vi "CreateExperimentRunNode.vi"(8 "Error In":errorcluster, 10 "Experiment Run":T1, 11 "DOM Document In":refnum<k20>) -> (0 "Error out":errorcluster, 2 "Experiment Run Node":refnum<k20>, 3 "DOM Document Out":refnum<k20>)   [LabVIEW 2012]
uses:
  ExperimentRun.ctl
  ExperimentRunTiming.ctl
  ExperimentRunDose.ctl
  ExperimentRunFluence.ctl
  ExperimentRunTotalCharge.ctl
  <resource>/objmgr/DOMUserDefRef.rc
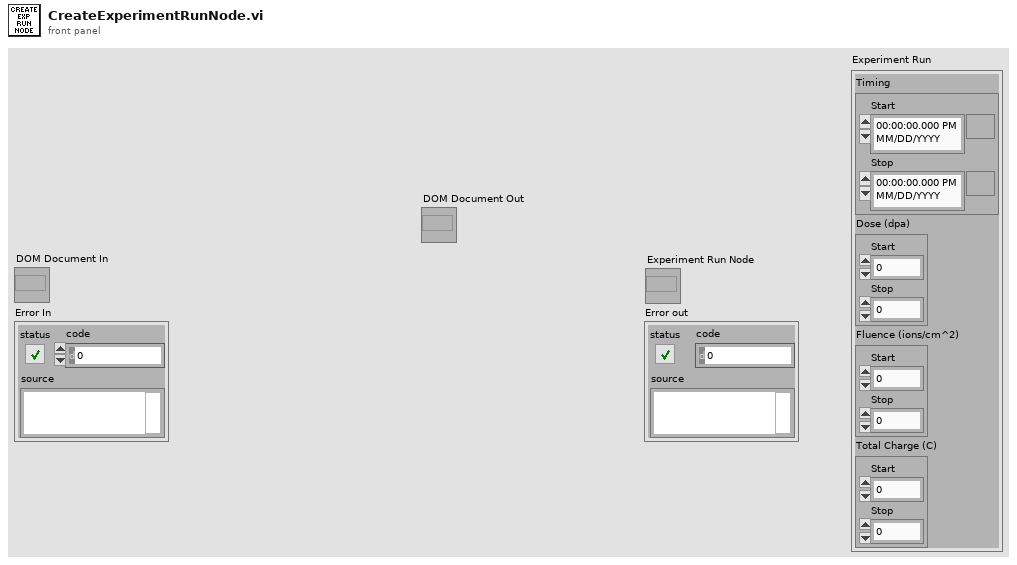
[diagram p1: front panel]
types:
  T1 = typedef "ExperimentRun.ctl" = cluster{"Timing":T2, "Dose (dpa)":T3, "Fluence (ions/cm^2)":T4, "Total Charge (C)":T5}
  T2 = typedef "ExperimentRunTiming.ctl" = cluster{"Start":timestamp, "Stop":timestamp}
  T3 = typedef "ExperimentRunDose.ctl" = cluster{"Start":dbl, "Stop":dbl}
  T4 = typedef "ExperimentRunFluence.ctl" = cluster{"Start":dbl, "Stop":dbl}
  T5 = typedef "ExperimentRunTotalCharge.ctl" = cluster{"Start":dbl, "Stop":dbl}
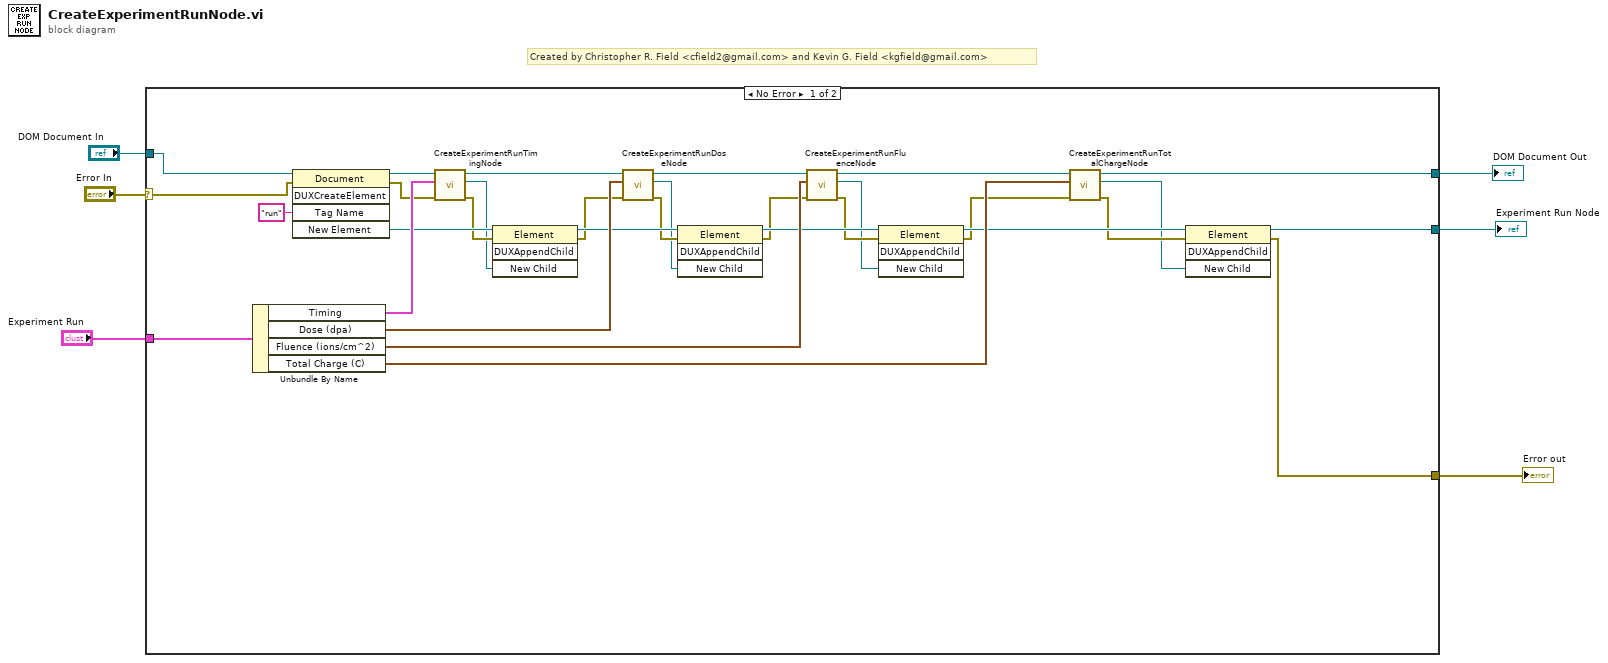
[diagram p0: block diagram]
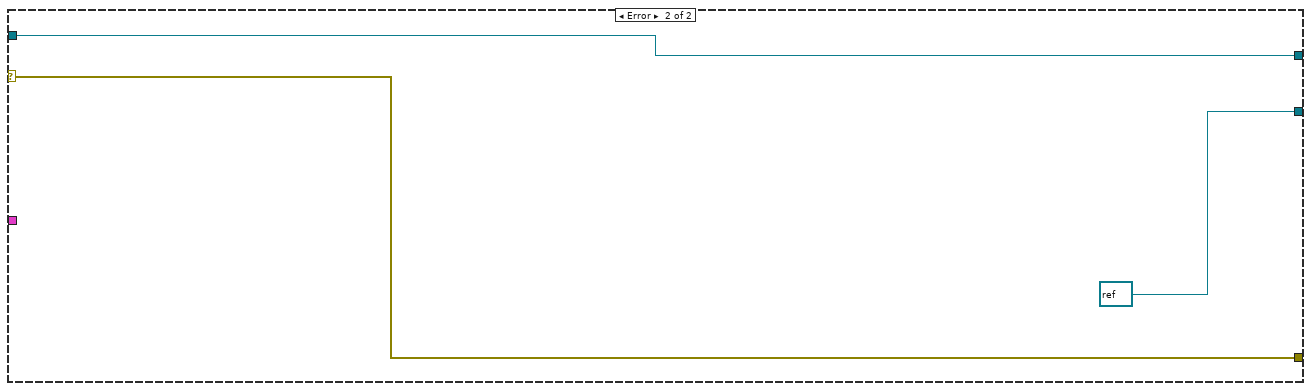
[diagram p2: hidden frame]
diagram:
  # "Created by Christopher R. Field <cfield2@gmail.com> and Kevin G. Field <kgfield@gmail.com>"
  n1 = case shown="No Error" "Error In" {
    selector: "Error In" -> [w35 w39]
    tunnel: "DOM Document In" -> [w37 w40]
    tunnel: [w19 refnum<k20> refnum ("Operator Node 2")] -> w5
    tunnel: [w18 w39] -> w4
    tunnel: [w21 w40] -> w2
    tunnel: "Experiment Run" -> [w34 _]
    frame No Error {
      n2 = Unbundle By Name(w34) -> ("Timing"=w32:T2, "Dose (dpa)"=w30:T3, "Fluence (ions/cm^2)"=w27:T4, "Total Charge (C)"=w25:T5)
      n3 = invoke class="Document" method="DUXCreateElement"(reference=w37, error in=w35, "Tag Name"="run") -> (reference out=w33:refnum<k20>, error out=w31:errorcluster, "New Element"=w24:refnum<k20>)  [unwired: 2 in, 2 out]
      n4 = call "CreateExperimentRunTimingNode.vi"("Error In"=w31, "Experiment Run Timing"=w32, "DOM Document In"=w33) -> ("Error out"=w17:errorcluster, "Experiment Run Timing Node"=w7:refnum<k20>, "DOM Document Out"=w29:refnum<k20>)  [unwired: 6 in]
      n5 = invoke class="Element" method="DUXAppendChild"(reference=w24, error in=w17, "New Child"=w7) -> (reference out=w23:refnum<k20>, error out=w16:errorcluster)  [unwired: 1 in, 2 out]
      n6 = call "CreateExperimentRunDoseNode.vi"("Error In"=w16, "Experiment Run Dose (dpa)"=w30, "DOM Document In"=w29) -> ("Error out"=w15:errorcluster, "Experiment Run Dose Node"=w8:refnum<k20>, "DOM Document Out"=w28:refnum<k20>)  [unwired: 6 in]
      n7 = invoke class="Element" method="DUXAppendChild"(reference=w23, error in=w15, "New Child"=w8) -> (reference out=w22:refnum<k20>, error out=w14:errorcluster)  [unwired: 1 in, 2 out]
      n8 = call "CreateExperimentRunFluenceNode.vi"("Error In"=w14, "Experiment Run Fluence (ions/cm^2)"=w27, "DOM Document In"=w28) -> ("Error out"=w13:errorcluster, "Experiment Run Fluence Node"=w9:refnum<k20>, "DOM Document Out"=w26:refnum<k20>)  [unwired: 6 in]
      n9 = invoke class="Element" method="DUXAppendChild"(reference=w22, error in=w13, "New Child"=w9) -> (reference out=w20:refnum<k20>, error out=w12:errorcluster)  [unwired: 1 in, 2 out]
      n10 = call "CreateExperimentRunTotalChargeNode.vi"("Error In"=w12, "Experiment Run Total Charge (C)"=w25, "DOM Document In"=w26) -> ("Error out"=w11:errorcluster, "Experiment Run Total Charge Node"=w10:refnum<k20>, "DOM Document Out"=w21:refnum<k20>)  [unwired: 6 in]
      n11 = invoke class="Element" method="DUXAppendChild"(reference=w20, error in=w11, "New Child"=w10) -> (reference out=w19:refnum<k20>, error out=w18:errorcluster)  [unwired: 1 in, 2 out]
    }
    frame Error {
    }
  }
  "Experiment Run Node" <- w5
  "Error out" <- w4
  "DOM Document Out" <- w2
